vi "ELVIS III v1.0 Read DIO.vi"(8 "error in (no error)":errorcluster, 10 "Channel List":T3, 11 "myRIO Ref In":T1) -> (0 "error out":errorcluster, 2 "bool Value List":bool[](array[boolean]), 3 "myRIO Ref Out":T1)   [LabVIEW 2021]
uses:
  <vilib>/myRIO/Common/Instrument Driver Framework/myRIO v1.0/DIO/typedefs/DIO Channels List.ctl
  <vilib>/myRIO/Common/Instrument Driver Framework/myRIO v1.0/DIO/typedefs/DIO Channels Enum.ctl
  <vilib>/myRIO/Common/Instrument Driver Framework/Utilities/typedefs/myRIO v1.0 Reference.ctl
  <vilib>/myRIO/Common/Instrument Driver Framework/Utilities/typedefs/Generic FPGA Reference.ctl
  <vilib>/myRIO/Common/Instrument Driver Framework/ELVIS III v1.0/DIO/typedefs/ELVIS III DIO FPGA Reference.ctl
  <vilib>/myRIO/Common/Instrument Driver Framework/ELVIS III v1.0/DIO/typedefs/ELVIS III DIO Bank Enum.ctl
  <vilib>/Utility/error.llb/Error Cluster From Error Code.vi
  <vilib>/rvi/errors/niLvFpgaAdjustHostInterfaceError.vi
  <vilib>/rvi/interface/nirviReadWriteControl/nirviReadWriteControl.xnode
  NiFpgaLv.dll
  <vilib>/rvi/interface/Simulation/niFpgaSimulationCallBeginRW.vi
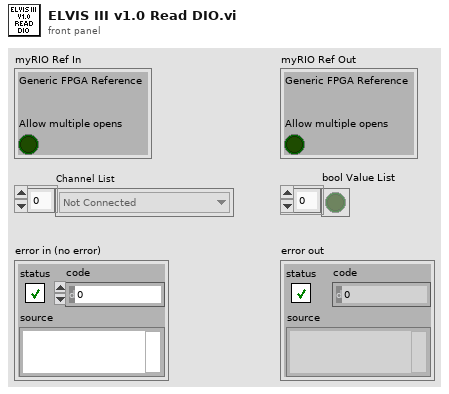
[diagram p1: front panel]
types:
  T1 = typedef "myRIO v1.0 Reference.ctl" = cluster{"Generic FPGA Reference":T2, "Allow multiple opens":bool}
  T2 = typedef "Generic FPGA Reference.ctl" = refnum<k20>
  T3 = typedef "DIO Channels List.ctl" = T4[]
  T4 = typedef "DIO Channels Enum.ctl" = enum16{"Not Connected", "C/DIO0", "C/DIO1", "C/DIO2", "C/DIO3", "C/DIO4", "C/DIO5", "C/DIO6", "C/DIO7", "A/DIO0", "A/DIO1", "A/DIO2", "A/DIO3", "A/DIO4", "A/DIO5", "A/DIO6", "A/DIO7", "A/DIO8", "A/DIO9", "A/DIO10", "A/DIO11", "A/DIO12", "A/DIO13", "A/DIO14", "A/DIO15", "A/DIO16", "A/DIO17", "A/DIO18", "A/DIO19", "B/DIO0", "B/DIO1", "B/DIO2", "B/DIO3", "B/DIO4", "B/DIO5", "B/DIO6", "B/DIO7", "B/DIO8", "B/DIO9", "B/DIO10", "B/DIO11", "B/DIO12", "B/DIO13", "B/DIO14", "B/DIO15", "B/DIO16", "B/DIO17", "B/DIO18", "B/DIO19", "LED0", "LED1", "LED2", "LED3", "Button0", "DIO/DIO0", "DIO/DIO1", "DIO/DIO2", "DIO/DIO3", "DIO/DIO4", "DIO/DIO5", "DIO/DIO6", "DIO/DIO7", "DIO/DIO8", "DIO/DIO9", "SPI/CS0", "SPI/CS1", "SPI/CS2", "SPI/CS3", "LED RADIO (Green)", "LED RADIO (Red)", "LED COMM (Green)", "LED COMM (Red)", "LED MODE (Green)", "LED MODE (Red)"}
  T5 = typedef "ELVIS III DIO Bank Enum.ctl" = enum32{"None", "A/DIO19:0", "B/DIO19:0", "LED3:0", "Button0"}
  T6 = typedef "ELVIS III DIO FPGA Reference.ctl" = refnum<k20>
  T7 = typedef "ELVIS III DIO Bitmask to Channel Map.ctl" = cluster{"DIO Bank Enum":T5, "Bit":i32}
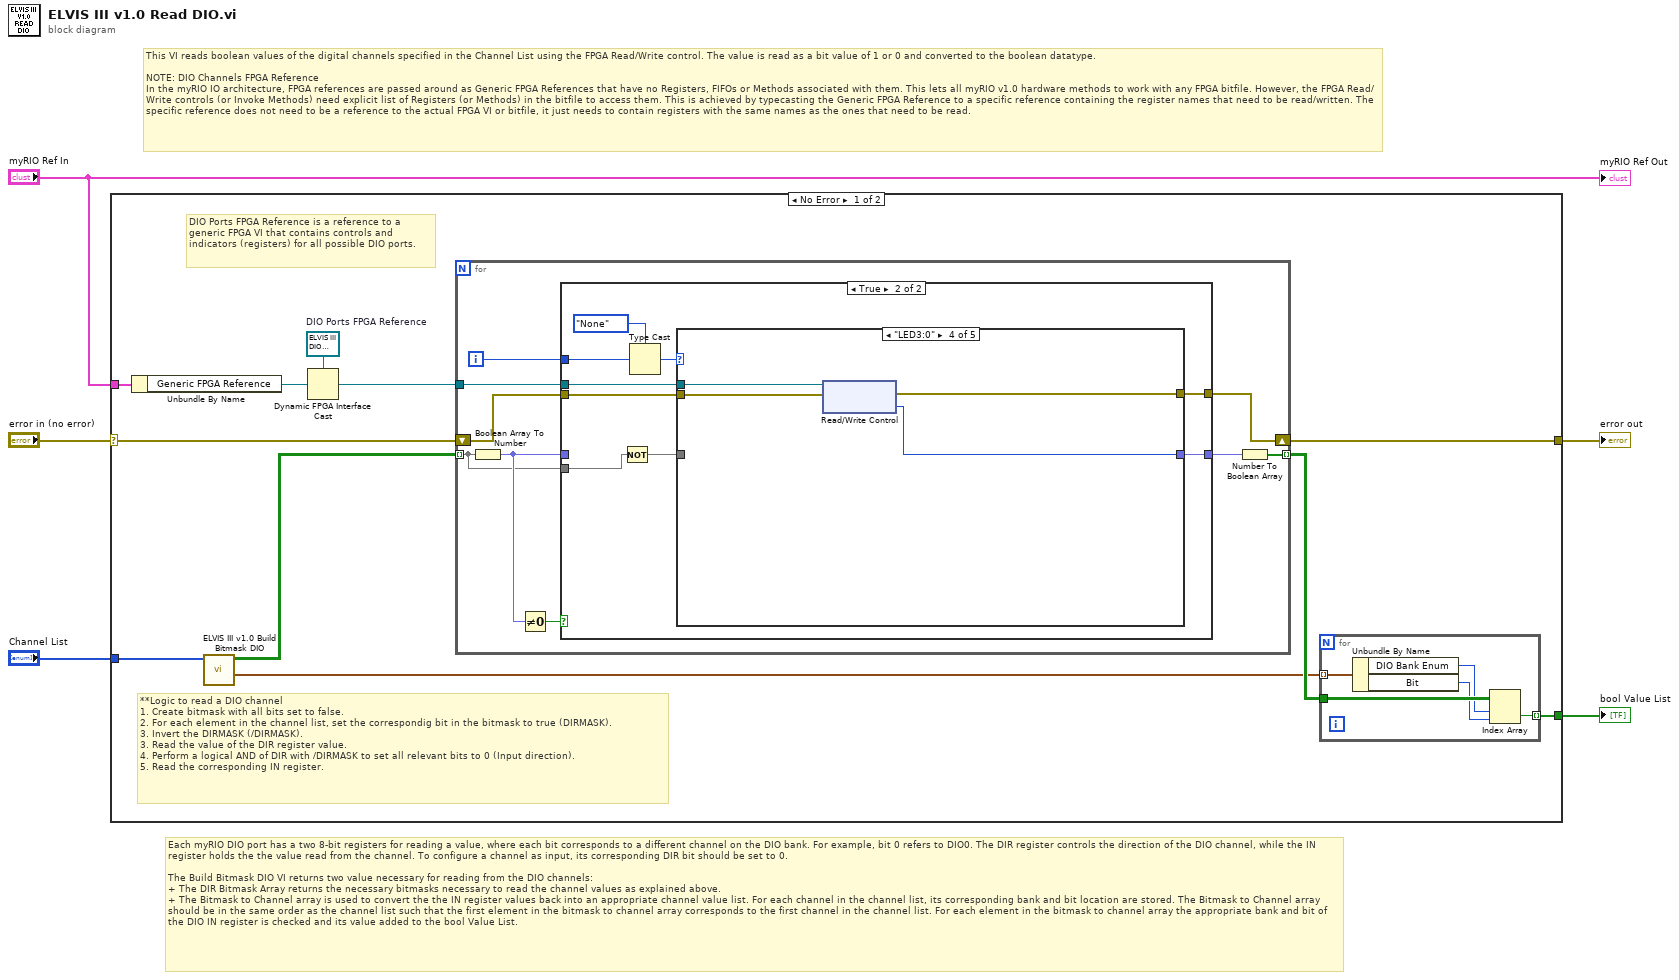
[diagram p0: block diagram]
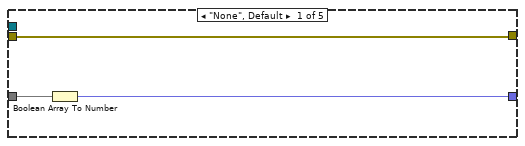
[diagram p3: hidden frame]
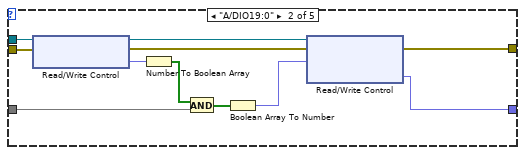
[diagram p4: hidden frame]
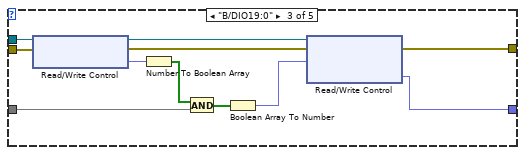
[diagram p5: hidden frame]
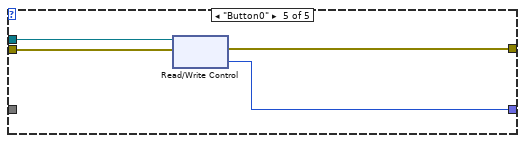
[diagram p6: hidden frame]
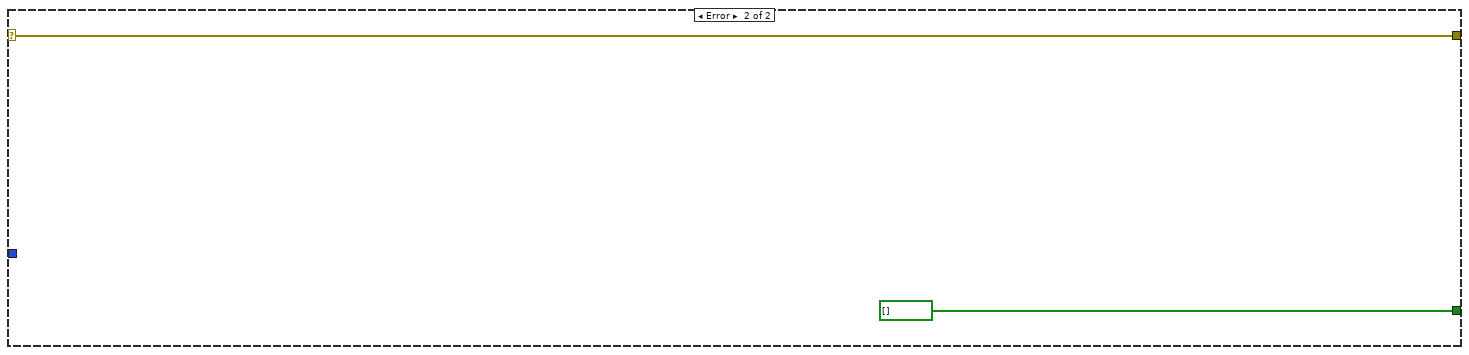
[diagram p7: hidden frame]
diagram:
  # "Each myRIO DIO port has a two 8-bit registers for reading a value, where each bit corresponds to a different channel on the DIO bank. For example, bit 0 refers to DIO0. The DIR register controls the direction of the DIO channel, while the IN register holds the the value read from the channel. To configure a channel as input, its corresponding DIR bit should be set to 0.\n\nThe Build Bitmask DIO VI returns two value necessary for reading from the DIO channels:\n+ The DIR Bitmask Array returns the necessary bitmasks necessary to read the channel values as explained above. \n+ The Bitmask to Channel array is used to convert the the IN register values back into an appropriate channel value list. For each channel in the channel list, its corresponding bank and bit location are stored. The Bitmask to Channel array should be in the same order as the channel list such that the first element in the bitmask to channel array corresponds to the first channel in the channel list. For each element in the bitmask to channel array the appropriate bank and bit of the DIO IN register is checked and its value added to the bool Value List."
  # "This VI reads boolean values of the digital channels specified in the Channel List using the FPGA Read/Write control. The value is read as a bit value of 1 or 0 and converted to the boolean datatype. \n\nNOTE: DIO Channels FPGA Reference\nIn the myRIO IO architecture, FPGA references are passed around as Generic FPGA References that have no Registers, FIFOs or Methods associated with them. This lets all myRIO v1.0 hardware methods to work with any FPGA bitfile. However, the FPGA Read/Write controls (or Invoke Methods) need explicit list of Registers (or Methods) in the bitfile to access them. This is achieved by typecasting the Generic FPGA Reference to a specific reference containing the register names that need to be read/written. The specific reference does not need to be a reference to the actual FPGA VI or bitfile, it just needs to contain registers with the same names as the ones that need to be read."
  n1 = case shown="No Error" "error in (no error)" {
    selector: "error in (no error)" -> [w7 w76]
    tunnel: "myRIO Ref In" -> [w13 _]
    tunnel: [w12 w76] -> w4
    tunnel: [w11 bool[] []] -> w2
    tunnel: "Channel List" -> [w10 _]
    frame No Error {
      w16 = T6 refnum  # DIO Ports FPGA Reference
      # "DIO Ports FPGA Reference is a reference to a generic FPGA VI that contains controls and indicators (registers) for all possible DIO ports."
      # "**Logic to read a DIO channel\n1. Create bitmask with all bits set to false.\n2. For each element in the channel list, set the correspondig bit in the bitmask to true (DIRMASK).\n3. Invert the DIRMASK (/DIRMASK).\n3. Read the value of the DIR register value.\n4. Perform a logical AND of DIR with /DIRMASK to set all relevant bits to 0 (Input direction).\n5. Read the corresponding IN register."
      n2 = Unbundle By Name(w13) -> ("Generic FPGA Reference"=w6:T2)
      n3 = call <vilib>:"ELVIS III v1.0 Build Bitmask DIO.vi"("Channel List"=w10) -> ("Bitmask to Channel Array"=w8:T7[], "DIR Bitmask Array"=w9:bool[][])  [unwired: 8 in, 1 out]
      n4 = Dynamic FPGA Interface Cast(Session In=w16, Type=w6) -> (Session Out=w15:T6)
      n5 = for {
        tunnel: w9 -> [w23] mode=indexing
        tunnel: w15 -> [w30]
        shift-right: [w28] -> w12
        shift-left: w7 -> [w27]
        tunnel: [w26] -> w14 mode=indexing
        i -> [w29]
        n6 = Boolean Array To Number(Boolean array=w23) -> (number=w24:fxp<+,20,20>)
        n7 = Not Equal To 0?(x=w24) -> (x != 0?=w25:bool)
        n8 = case shown="True" w25 {
          tunnel: w30 -> [_ w41]
          tunnel: w29 -> [_ w40]
          tunnel: w24 -> [w31 _]
          tunnel: [w32 w36] -> w28
          tunnel: w27 -> [w32 w35]
          tunnel: w23 -> [_ w34]
          tunnel: [w31 w33] -> w22
          frame False {
          }
          frame True {
            n9 = Not(x=w34) -> (.not. x?=w37:bool[])
            n10 = Type Cast(type=ELVIS_III_DIO_Bank_Enum."None" ("DIO Bank Enum"), x=w40) -> (*(type *) &x=w38:T5)
            n11 = case shown="\"LED3:0\"" w38 {
              tunnel: w41 -> [_ w55 w66 w70 w74]
              tunnel: w37 -> [w43 w51 w62 _ _]
              tunnel: [w44 w45 w56 w68 w72] -> w36
              tunnel: w35 -> [w44 w47 w58 w69 w73]
              tunnel: [w42 w48 w59 w67 w71] -> w33
              frame "None", Default {
                n12 = Boolean Array To Number(Boolean array=w43) -> (number=w42:fxp<+,20,20>)
              }
              frame "A/DIO19:0" {
                n13 = xnode "Read/Write Control"("FPGA VI Reference In"=w55, "error in"=w47) -> ("FPGA VI Reference Out"=w54:T6, "error out"=w46:errorcluster, "DIO.A_19:0.DIR"=w53:fxp<+,20,20>)
                n14 = Number To Boolean Array(number=w53) -> (Boolean array=w52:bool[])
                n15 = And(x=w52, y=w51) -> (x .and. y?=w50:bool[])
                n16 = Boolean Array To Number(Boolean array=w50) -> (number=w49:fxp<+,20,20>)
                n17 = xnode "Read/Write Control"("FPGA VI Reference In"=w54, "error in"=w46, "DIO.A_19:0.DIR"=w49) -> ("error out"=w45:errorcluster, "DIO.A_19:0.IN"=w48:fxp<+,20,20>)  [unwired: 1 out]
              }
              frame "B/DIO19:0" {
                n18 = xnode "Read/Write Control"("FPGA VI Reference In"=w66, "error in"=w58) -> ("FPGA VI Reference Out"=w65:T6, "error out"=w57:errorcluster, "DIO.B_19:0.DIR"=w64:fxp<+,20,20>)
                n19 = Number To Boolean Array(number=w64) -> (Boolean array=w63:bool[])
                n20 = And(x=w63, y=w62) -> (x .and. y?=w61:bool[])
                n21 = Boolean Array To Number(Boolean array=w61) -> (number=w60:fxp<+,20,20>)
                n22 = xnode "Read/Write Control"("FPGA VI Reference In"=w65, "error in"=w57, "DIO.B_19:0.DIR"=w60) -> ("error out"=w56:errorcluster, "DIO.B_19:0.IN"=w59:fxp<+,20,20>)  [unwired: 1 out]
              }
              frame "LED3:0" {
                n23 = xnode "Read/Write Control"("FPGA VI Reference In"=w70, "error in"=w69) -> ("error out"=w68:errorcluster, "DO.LED3:0"=w67:u8)  [unwired: 1 out]
              }
              frame "Button0" {
                n24 = xnode "Read/Write Control"("FPGA VI Reference In"=w74, "error in"=w73) -> ("error out"=w72:errorcluster, "DI.BTN"=w71:u8)  [unwired: 1 out]
              }
            }
          }
        }
        n25 = Number To Boolean Array(number=w22) -> (Boolean array=w26:bool[])
      }
      n26 = for {
        tunnel: [w18] -> w11 mode=indexing
        tunnel: w14 -> [w21]
        tunnel: w8 -> [w17] mode=indexing
        n27 = Unbundle By Name(w17) -> ("DIO Bank Enum"=w20:T5, "Bit"=w19:i32)
        n28 = Index Array(array=w21, index (row)=w20, index (col)=w19) -> (element=w18:bool)
      }
    }
    frame Error {
    }
  }
  "error out" <- w4
  "bool Value List" <- w2
  "myRIO Ref Out" <- "myRIO Ref In"
